vi "UiCharts24h_b2g1.vi"() -> ()   [LabVIEW 2011]
uses:
  Output - Cluster b2g1.ctl
  Input - Cluster b2g1.ctl
  <vilib>/Platform/TimedLoop/XDataNode/timing_clust.ctl
  <vilib>/Platform/TimedLoop/XDataNode/nitl_modes.ctl
  <vilib>/Platform/TimedLoop/XDataNode/wakeup.ctl
  <vilib>/addons/database/Connection.llb/DB Tools Open Connec (String).vi
  <vilib>/addons/database/Connection.llb/Conn Execute.vi
  <vilib>/addons/database/Recordset.llb/Rec Fetch Recordset Data (R).vi
  <vilib>/addons/database/Recordset.llb/Rec Destroy - Connection.vi
  <vilib>/Platform/TimedLoop/XDataNode/XDataNode.xnode
  <vilib>/addons/database/_DB Variant To Data/Database Variant To Data.xnode
  <vilib>/Platform/TimedLoop/XDataNode/XDNodeRunTimeDep.lvlib
  <vilib>/addons/database/NI_Database_API.lvlib
panel:
  in  "Output Var":refnum<k21>="ni.var.psp://10.27.40.24/variables - b2g1/data - network - b2g1"
  in  "Input Var":refnum<k21>="ni.var.psp://10.27.40.24/variables - b2g1/input - network b2g1"
  in  "Tab Control":T1(tab)
  out "protocol":string[][](table)
  out "pH-Wert":dbl(graph)
  out "Temperaturregelung":T2(graph)
  out "Füllstandsregelung":T3(graph)
  out "Druckregelung":T4(graph)
  out "error out":errorcluster
  in  "stop":bool
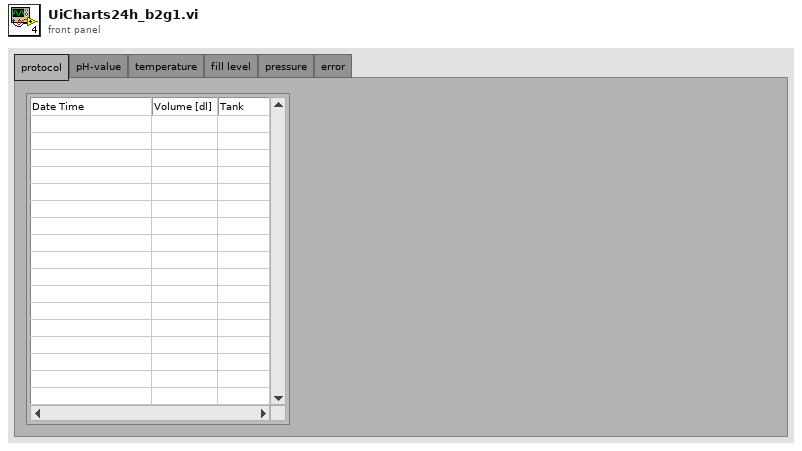
[diagram p1: front panel]
types:
  T1 = enum32{"protocol", "pH-value", "temperature", "fill level", "pressure", "error"}
  T2 = cluster{"Temp Soll [°C]":sgl, "TS-4 [°C]":dbl, dbl, dbl}
  T3 = cluster{"Füllstand Soll [l]":sgl, "FS-3 [l]":dbl, dbl}
  T4 = cluster{"Druck Soll [bar]":sgl, "DS-1 [bar]":dbl, dbl, dbl}
  T5 = typedef "Input - Cluster b2g1.ctl" = cluster{"V-13 [%]":u8, "V-15 [%]":u8, "Log-Target":bool, "P-4":bool, "P-4 Drehzahl [%]":u8, "Temperaturregelung":bool, "Überdruckregelung":bool, "Füllstandsregulierung":bool, "V-10":bool, "Log-Host":bool, "V-14":bool, "P-5":bool, "P-5 Drehzahl [%]":u8, "HS-1":bool, "Füllstand  P":sgl, "Füllstand I":sgl, "Füllstand D":sgl, "Füllstand Soll [l]":sgl, "Druck  P":sgl, "Druck I":sgl, "Druck D":sgl, "Druck Soll [bar]":sgl, "Temp Soll [°C]":sgl, "Dosierung":bool, "Dosiermenge [l]":sgl, "Dosiergeschw. [l/min]":sgl, "Tank":bool, "Hysterese [°C]":sgl, "MR Füllstandsüberwachung":bool, "Tank Füllstandsüberwachung":bool, "Log Target [ms]":u32, "Log Host [s]":u32, "P-5 EIN [min]":u8, "P-5 AUS [min]":u8, "Zirkulation":bool, "V-33":bool, "V-34":bool}
  T6 = typedef "Output - Cluster b2g1.ctl" = cluster{"DFS-1 [dl]":u64, "FS-3 [l]":dbl, "DFS-1 [l/min]":dbl, "DS-1 [bar]":dbl, "V-10 ZU":bool, "V-14 ZU":bool, "FS-1 [l]":dbl, "FS-2 [l]":dbl, "TS-4 [°C]":dbl, "HS-1":bool, "V-13 [%]":u8, "V-15 [%]":u8, "P-4 [%]":u8, "P-5 [%]":u8, "Dosierung":bool, "MR Max Füllstand":bool, "MR Min Füllstand":bool, "Dosiermenge [l]":sgl, "V-14 AUF":bool, "V-10 AUF":bool, "T-1 Max Füllstand":bool, "T-1 Min Füllstand":bool, "T-2 Max Füllstand":bool, "T-2 Min Füllstand":bool, "pHS-1 [pH]":dbl, "P-4 RUN":bool, "P-5 RUN ":bool, "V-33 AUF":bool, "V-33 ZU":bool, "V-34 AUF":bool, "V-34 ZU":bool, "P-4 ERR":bool, "P-5 ERR":bool, "TS-5 [°C]":dbl, "GZ-1 [dl]":u64, "TS-6 [°C]":dbl, "DS-3 [bar]":dbl}
  T7 = typedef "XDNodeRunTimeDep.lvlib/timing_clust.ctl" = cluster{"Expected End [f-1]":u64, "Actual End [f-1]":u64, "Finished Late? [f-1]":bool, "Expected End [i-1]":u64, "Actual End [i-1]":u64, "Finished Late? [i-1]":bool, "Expected Start [i]":u64, "Actual Start [i]":u64, "Expected Start [f]":u64, "Actual Start [f]":u64, "Source Name":string, "Structure Name":string, "Period":i64, "Deadline":i64, "Offset":i64, "Start":i64, "Priority":i32, "Timeout":i32, "Mode":T8, "Wakeup Reason":T9, "Error":errorcluster, "Source Type":string, "Secondary Source Type":string, "Global End Time":u64, "Global Start Time":u64, "Frame Duration":u64, "Iteration Duration":u64, "Assigned CPU":i32, "I/O Scan Engine Mode":u32}
  T8 = typedef "XDNodeRunTimeDep.lvlib/nitl_modes.ctl" = enum32{"No Change", "Process missed periods, maintain original phase", "Discard missed periods, maintain original phase", "Process missed periods, ignore original phase", "Discard missed periods, ignore original phase"}
  T9 = typedef "XDNodeRunTimeDep.lvlib/wakeup.ctl" = enum32{"Normal", "Aborted", "Asynchronous wakeup", "Timing source error", "Timed loop error", "Timeout"}
  T10 = typedef "NI_Database_API.lvlib/Conn ObjectReference.ctl" = refnum<k1>
  T11 = typedef "NI_Database_API.lvlib/Rec ObjectReference.ctl" = refnum<k1>
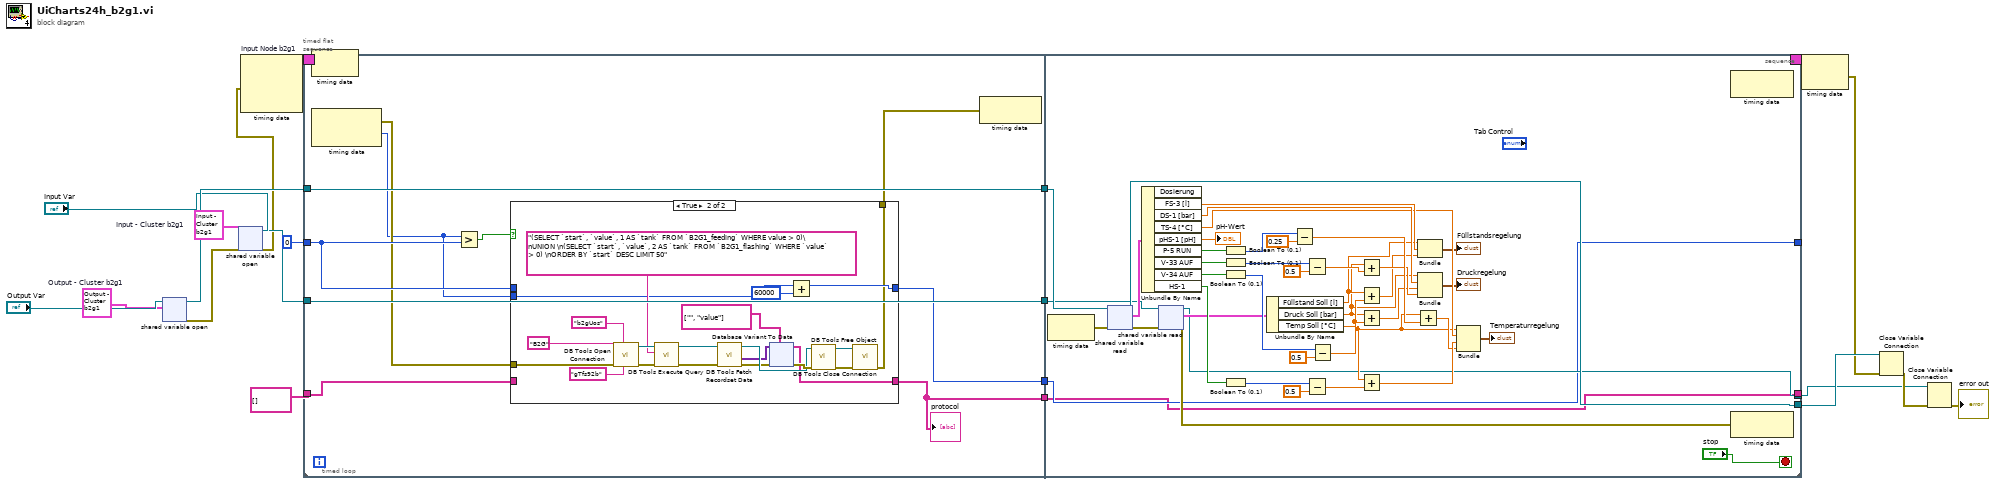
[diagram p0: block diagram]
diagram:
  w12 = T5 {"V-13 [%]"=0, "V-15 [%]"=0, "Log-Target"=FALSE, "P-4"=FALSE, "P-4 Drehzahl [%]"=0, "Temperaturregelung"=FALSE, "Überdruckregelung"=FALSE, "Füllstandsregulierung"=FALSE, "V-10"=FALSE, "Log-Host"=FALSE, "V-14"=FALSE, "P-5"=FALSE, "P-5 Drehzahl [%]"=0, "HS-1"=FALSE, "Füllstand  P"=0.0, "Füllstand I"=0.0, "Füllstand D"=0.0, "Füllstand Soll [l]"=0.0, "Druck  P"=0.0, "Druck I"=0.0, "Druck D"=0.0, "Druck Soll [bar]"=0.0, "Temp Soll [°C]"=0.0, "Dosierung"=FALSE, "Dosiermenge [l]"=0.0, "Dosiergeschw. [l/min]"=0.0, "Tank"=FALSE, "Hysterese [°C]"=0.0, "MR Füllstandsüberwachung"=FALSE, "Tank Füllstandsüberwachung"=FALSE, "Log Target [ms]"=0, "Log Host [s]"=0, "P-5 EIN [min]"=0, "P-5 AUS [min]"=0, "Zirkulation"=FALSE, "V-33"=FALSE, "V-34"=FALSE}  # Input - Cluster b2g1
  w16 = T6 {"DFS-1 [dl]"=0, "FS-3 [l]"=0.0, "DFS-1 [l/min]"=0.0, "DS-1 [bar]"=0.0, "V-10 ZU"=FALSE, "V-14 ZU"=FALSE, "FS-1 [l]"=0.0, "FS-2 [l]"=0.0, "TS-4 [°C]"=0.0, "HS-1"=FALSE, "V-13 [%]"=0, "V-15 [%]"=0, "P-4 [%]"=0, "P-5 [%]"=0, "Dosierung"=FALSE, "MR Max Füllstand"=FALSE, "MR Min Füllstand"=FALSE, "Dosiermenge [l]"=0.0, "V-14 AUF"=FALSE, "V-10 AUF"=FALSE, "T-1 Max Füllstand"=FALSE, "T-1 Min Füllstand"=FALSE, "T-2 Max Füllstand"=FALSE, "T-2 Min Füllstand"=FALSE, "pHS-1 [pH]"=0.0, "P-4 RUN"=FALSE, "P-5 RUN "=FALSE, "V-33 AUF"=FALSE, "V-33 ZU"=FALSE, "V-34 AUF"=FALSE, "V-34 ZU"=FALSE, "P-4 ERR"=FALSE, "P-5 ERR"=FALSE, "TS-5 [°C]"=0.0, "GZ-1 [dl]"=0, "TS-6 [°C]"=0.0, "DS-3 [bar]"=0.0}  # Output - Cluster b2g1
  n1 = shared-variable-open("Output Var", w16) -> (w15:refnum<k21>, w9:errorcluster)  [unwired: 2 in]
  n2 = shared-variable-open("Input Var", w9, w12) -> (w10:refnum<k21>, w8:errorcluster)  [unwired: 1 in]
  n3 = node-c288 "Input Node b2g1"(w8) -> (w2:T7)  [unwired: 2 in]
  n4 = timed-loop {
    timing: w2 -> [_]
    timing-out: [_] -> w1
    tunnel: w15 -> [w25]
    tunnel: [w24] -> w14
    tunnel: w10 -> [w23]
    tunnel: [w22] -> w6
    tunnel: i64 0 -> [w21]
    tunnel: [w20] -> _
    tunnel: string[][] [] ("data") -> [w19]
    tunnel: [w18] -> _
    stop <- "stop" stop-if-true
    n5 = timed-sequence {
      timing: _ -> [_]
      timing-out: _ -> [_]
      tunnel: w25 -> [w37]
      tunnel: [w36] -> w24
      tunnel: w23 -> [w35]
      tunnel: [w34] -> w22
      tunnel: w21 -> [w29]
      tunnel: [w28] -> w20
      tunnel: w19 -> [w27]
      tunnel: [w26] -> w18
      n6 = timed-flat-sequence {
        tunnel: w35 -> [w46]
        tunnel: w37 -> [w47]
        tunnel: [w47] -> w33
        tunnel: [w46] -> w32
        tunnel: [w44] -> w31
        tunnel: [w42] -> w30
        tunnel: w29 -> [w43]
        tunnel: w27 -> [w41]
        tunnel: [w163] -> w36
        tunnel: [w125] -> w34
        tunnel: w33 -> [w164]
        tunnel: w32 -> [w130]
        tunnel: w31 -> [w124]
        tunnel: w30 -> [w123]
        tunnel: [w124] -> w28
        tunnel: [w123] -> w26
        frame #0 {
          n7 = node-c288() -> (w40:errorcluster, w38:i64)  [unwired: 1 in]
          n8 = Greater?(x=w38, y=w43) -> (0:w45:bool)
          n9 = case shown="True" w45 {
            tunnel: [w49 w59] -> w42
            tunnel: [w50 w57] -> w44
            tunnel: w43 -> [w50 _]
            tunnel: w38 -> [_ w58]
            tunnel: w41 -> [w49 _]
            tunnel: w40 -> [w48 w55]
            tunnel: [w48 w54] -> w39
            frame False {
            }
            frame True {
              n10 = call-poly <vilib>:"DB Tools Open Connection.vi"("password"="gTfs92b", "userID"="b2gUos", "error in (no error)"=w55, "connection information"="B2G") -> ("error out"=w66:errorcluster, "connection reference"=w67:T10)  [unwired: 4 in]
              n11 = call-poly <vilib>:"DB Tools Execute Query.vi"("error in (no error)"=w66, "SQL query"="(SELECT `start`, `value`, 1 AS `tank` FROM `B2G1_feeding` WHERE value > 0)\nUNION \n(SELECT `start`, `value`, 2 AS `tank` FROM `B2G1_flashing` WHERE `value` > 0) \nORDER BY `start` DESC LIMIT 50", "connection reference"=w67) -> ("error out"=w63:errorcluster, "recordset reference"=w61:T11)  [unwired: 5 in]
              n12 = call-poly <vilib>:"DB Tools Fetch Recordset Data.vi"("error in (no error)"=w63, "recordset reference"=w61) -> ("error out"=w64:errorcluster, "recordset data"=w65:variant[][], "recordset reference out"=w68:T11)  [unwired: 3 in]
              n13 = xnode "Database Variant To Data"("database variant"=w65, "error in"=w64, "type"=string[][] [["", "value"]] ("columns")) -> ("data"=w59:string[][], "error out"=w70:errorcluster)
              n14 = Add(x=w58, y=i64 60000) -> (x+y=w57:i64)
              n15 = call-poly <vilib>:"DB Tools Free Object.vi"("error in (no error)"=w70, "recordset reference"=w68) -> ("error out"=w71:errorcluster, "connection reference"=w69:T10)  [unwired: 8 in]
              n16 = call <vilib>:"DB Tools Close Connection.vi"("error in (no error)"=w71, "connection reference"=w69) -> ("error out"=w54:errorcluster)  [unwired: 5 in]
            }
          }
          "protocol" <- w42
          n17 = node-c288(w39) -> ()  [unwired: 1 out]
        }
        frame #1 {
          n18 = node-c288() -> (w133:errorcluster)  [unwired: 1 in]
          n19 = shared-variable-read(w164, w133) -> (w163:refnum<k21>, w132:errorcluster, w162:T6)  [unwired: 1 out]
          n20 = Unbundle By Name(w162) -> ("FS-3 [l]"=w161:dbl, "DS-1 [bar]"=w160:dbl, "TS-4 [°C]"=w159:dbl, "pHS-1 [pH]"=→"pH-Wert":dbl, "P-5 RUN"=w155:bool, "V-33 AUF"=w157:bool, "V-34 AUF"=w156:bool, "HS-1"=w154:bool)  [unwired: 1 out]
          n21 = shared-variable-read(w130, w132) -> (w125:refnum<k21>, w131:errorcluster, w129:T5)  [unwired: 1 out]
          n22 = Boolean To (0,1)(Boolean=w155) -> (0, 1=w147:i16)
          n23 = Boolean To (0,1)(Boolean=w157) -> (0, 1=w138:i16)
          n24 = Boolean To (0,1)(Boolean=w156) -> (0, 1=w137:i16)
          n25 = Boolean To (0,1)(Boolean=w154) -> (0, 1=w150:i16)
          n26 = Unbundle By Name(w129) -> ("Füllstand Soll [l]"=w128:sgl, "Druck Soll [bar]"=w126:sgl, "Temp Soll [°C]"=w127:sgl)
          n27 = Subtract(x=w147, y=0.25) -> (x-y=w149:dbl)
          n28 = Subtract(x=w138, y=0.5) -> (x-y=w145:dbl)
          n29 = Subtract(x=w150, y=0.5) -> (x-y=w153:dbl)
          n30 = Subtract(x=w137, y=0.5) -> (x-y=w139:dbl)
          n31 = Add(x=w126, y=w145) -> (x+y=w143:dbl)
          n32 = Add(x=w128, y=w139) -> (x+y=w140:dbl)
          n33 = Add(x=w126, y=w139) -> (x+y=w141:dbl)
          n34 = Add(x=w127, y=w153) -> (x+y=w152:dbl)
          n35 = Add(x=w127, y=w149) -> (x+y=w146:dbl)
          n36 = Bundle("Füllstand Soll [l]"=w128, "FS-3 [l]"=w161, w140) -> (→"Füllstandsregelung":T3)  [unwired: 1 in]
          n37 = Bundle("Druck Soll [bar]"=w126, "DS-1 [bar]"=w160, w141, w143) -> (→"Druckregelung":T4)  [unwired: 1 in]
          n38 = Bundle("Temp Soll [°C]"=w127, "TS-4 [°C]"=w159, w152, w146) -> (→"Temperaturregelung":T2)  [unwired: 1 in]
          n39 = node-c288(w131) -> ()  [unwired: 1 out]
        }
      }
    }
    n40 = node-c288() -> ()  [unwired: 1 in, 1 out]
    n41 = node-c288() -> ()  [unwired: 1 in, 1 out]
  }
  n42 = node-c288(w1) -> (w13:errorcluster)
  n43 = Close Variable Connection(8:w13, 11:w14) -> (0:w7:errorcluster)
  n44 = Close Variable Connection(8:w7, 11:w6) -> (0:→"error out":errorcluster)
